vi "Config TDMS File for Asynchronous Write.vi"(8 "error in (no error)":errorcluster, 10 "rx channels":T1={"rx config"={"channel configuration"=[], "transfer mode"=enum."Finite", "sample rate"=10000000.0, "number of samples"=8192, "start trigger"=enum."Immediate"}, "reference frequency source"="Internal", "rx.data sink"=enum."Host", "rx.enabled channels"=[], "vertical range"=[], "rx.coerced configurations"={"coerced frequencies"=[], "coerced lo frequencies"=[], "coerced levels"=[], "coerced sample rates"=[]}} {"rx.coerced configurations"."coerced sample rates" format="%#.3pS/s"; "rx.coerced configurations"."coerced levels" format="%#.3gdBm"; "rx.coerced configurations"."coerced lo frequencies" format="%#.3pHz"; "rx.coerced configurations"."coerced frequencies" format="%#.3pHz"; "rx config"."channel configuration"."channel configuration"."frequency" format="%#.3pHz"; "rx config"."channel configuration"."channel configuration"."lo frequency" format="%#.3pHz"; "rx config"."channel configuration"."channel configuration"."level" format="%#_gdBm"; "rx config"."sample rate" format="%#.3pS/s"; "vertical range" format="%#.3pVpp"}, 11 "base path":path=path "D:/USRP Project TDMS Files") -> (0 "error out":errorcluster, 3 "Refnums out":refnum<k34>[](array[refnum]))   [LabVIEW 2016]
doc: "Configure TDMS Settings for asynchronous write"
uses:
  2954/SubVIs/Rx Channels.ctl
  2954/SubVIs/Start Trigger.ctl
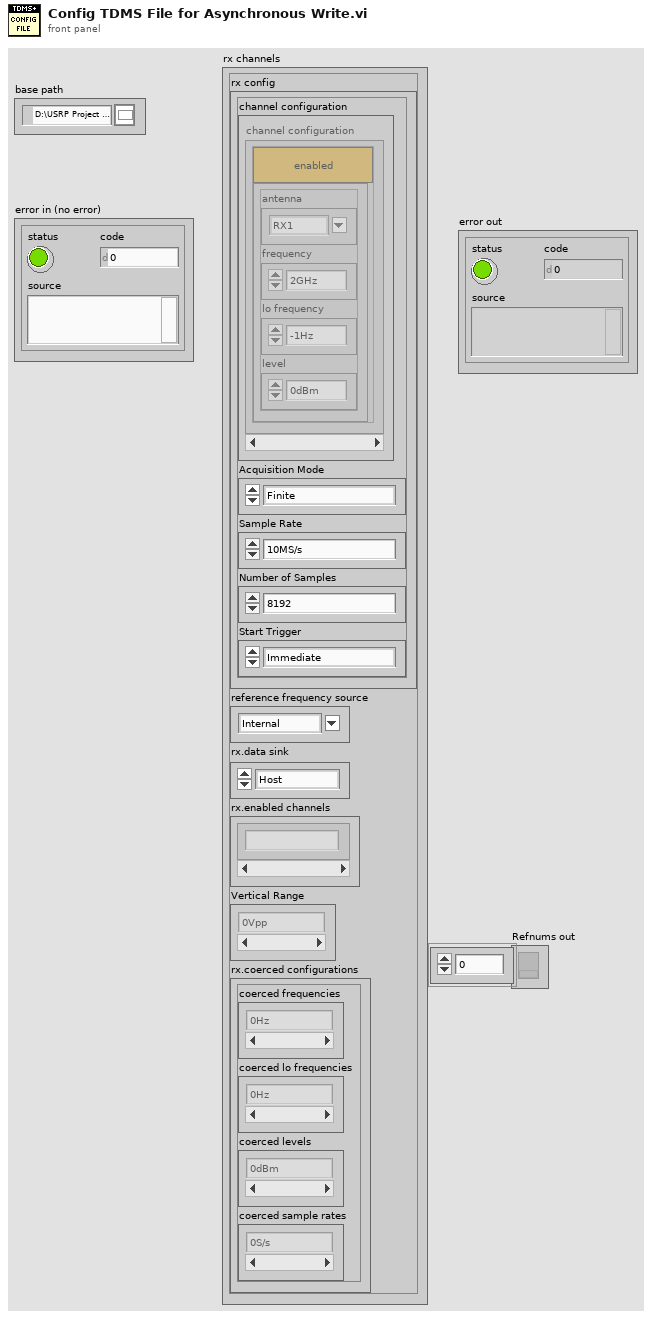
[diagram p1: front panel]
types:
  T1 = typedef "Rx Channels.ctl" = cluster{"rx config":cluster{"channel configuration":cluster{"channel enable":bool, "channel configuration":cluster{"antenna":string, "frequency":dbl, "lo frequency":dbl, "level":dbl}}[], "transfer mode":enum16{"Finite", "Continuous"}, "sample rate":dbl, "number of samples":u32, "start trigger":T2}, "reference frequency source":string, "rx.data sink":enum16{"SFP Port 0", "SFP Port 1", "Host"}, "rx.enabled channels":string[], "vertical range":dbl[], "rx.coerced configurations":cluster{"coerced frequencies":dbl[], "coerced lo frequencies":dbl[], "coerced levels":dbl[], "coerced sample rates":dbl[]}}
  T2 = typedef "Start Trigger.ctl" = enum8{"Software", "Digital Edge", "Rx Start Trigger", "Tx Start Trigger", "Immediate", "Future Time Event"}
  T3 = enum16{"open", "open or create", "create or replace", "create", "open (read-only)"}
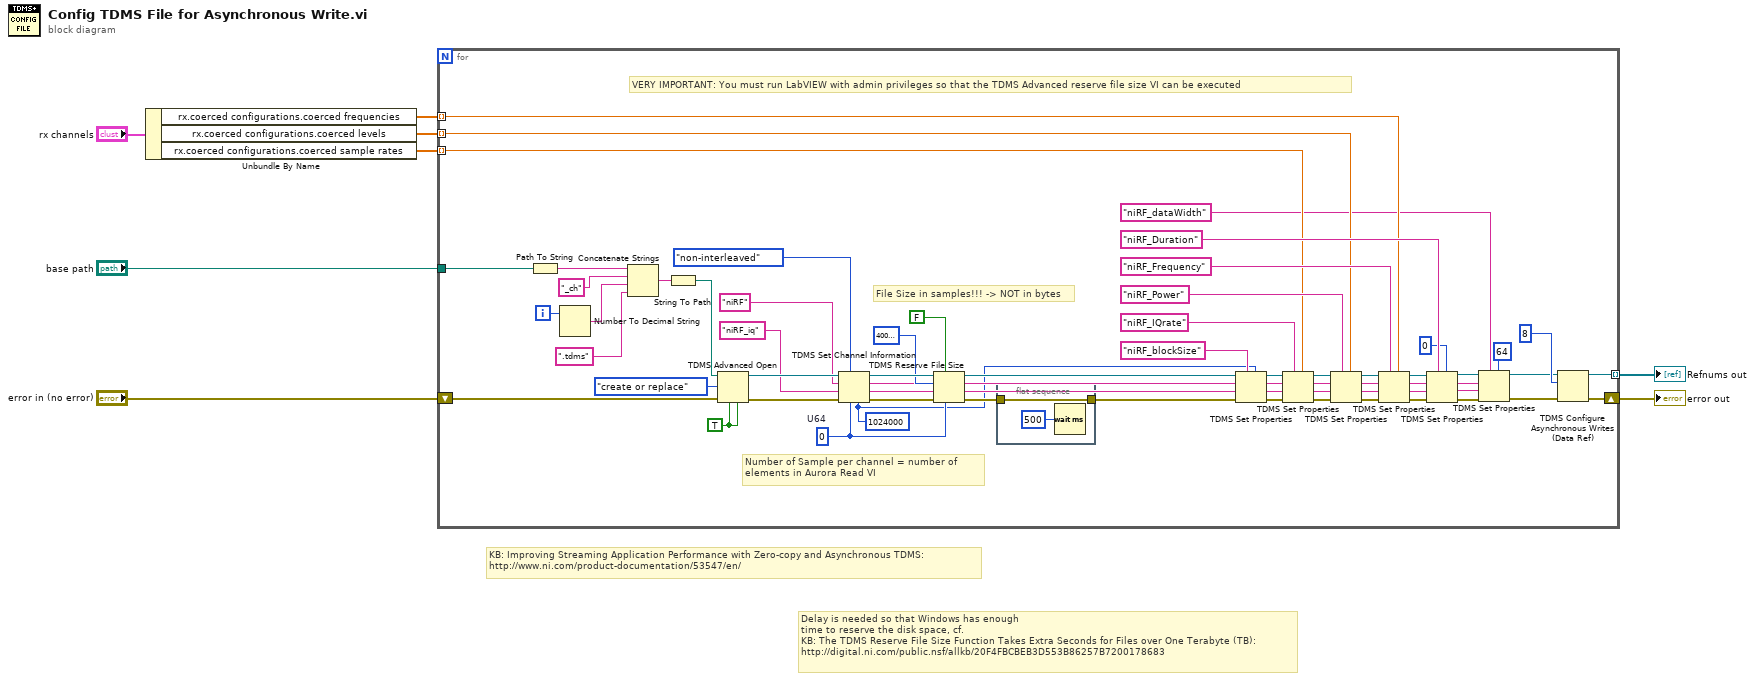
[diagram p0: block diagram]
diagram:
  # "KB: Improving Streaming Application Performance with Zero-copy and Asynchronous TDMS:\nhttp://www.ni.com/product-documentation/53547/en/"
  # "Delay is needed so that Windows has enough \ntime to reserve the disk space, cf.\nKB: The TDMS Reserve File Size Function Takes Extra Seconds for Files over One Terabyte (TB): \nhttp://digital.ni.com/public.nsf/allkb/20F4FBCBEB3D553B86257B7200178683"
  n1 = Unbundle By Name("rx channels") -> ("rx.coerced configurations.coerced frequencies"=w5:dbl[], "rx.coerced configurations.coerced levels"=w4:dbl[], "rx.coerced configurations.coerced sample rates"=w3:dbl[])
  n2 = for {
    shift-right: [w68] -> w8
    shift-left: "error in (no error)" -> [w60]
    tunnel: w5 -> [w32] mode=indexing
    tunnel: w4 -> [w31] mode=indexing
    tunnel: w3 -> [w30] mode=indexing
    tunnel: "base path" -> [w15]
    tunnel: [w11] -> w1 mode=indexing
    i -> [w13]
    w34 = "niRF_iq"
    w35 = "niRF"
    w20 = u32 1024000 ("samples per channel")
    w67 = u64 0  # U64
    w66 = TRUE ("enable asynchronous? (T)")
    # "File Size in samples!!! -> NOT in bytes"
    # "VERY IMPORTANT: You must run LabVIEW with admin privileges so that the TDMS Advanced reserve file size VI can be executed"
    # "Number of Sample per channel = number of \nelements in Aurora Read VI"
    n3 = Path To String(path=w15) -> (string=w16:string)
    n4 = Number To Decimal String(number=w13) -> (decimal integer string=w14:string)  [unwired: 1 in]
    n5 = Concatenate Strings(w16, "_ch" ("string"), w14, ".tdms" ("string")) -> (w18:string)
    n6 = String To Path(string=w18) -> (path=w12:path)
    n7 = TDMS Advanced Open(4:w66, 6:w66, 8:w60, 10:T3."create or replace" ("operation (0:open)"), 11:w12) -> (0:w61:errorcluster, 3:w62:refnum<k34>)  [unwired: 1 out]
    n8 = TDMS Set Channel Information(4:w20, 6:w67, 7:enum16{"non-interleaved", "interleaved"}."non-interleaved" ("data layout (0:non-interleaved)"), 8:w61, 9:w34, 10:w35, 11:w62) -> (0:w64:errorcluster, 3:w65:refnum<k34>)
    n9 = TDMS Reserve File Size(6:w67, 7:FALSE ("append? (T)"), 8:w64, 10:u64 40000000000 ("reserve size"), 11:w65) -> (0:w58:errorcluster, 3:w44:refnum<k34>)
    n10 = flat-sequence {
      tunnel: w58 -> [w71]
      tunnel: [w71] -> w33
      frame #0 {
        n11 = Wait (ms)(milliseconds to wait=u32 500) -> ()  [unwired: 1 out]
      }
    }
    n12 = TDMS Set Properties(5:w20, 7:"niRF_blockSize", 8:w33, 9:w34, 10:w35, 11:w44) -> (0:w42:errorcluster, 1:w40:string, 2:w41:string, 3:w43:refnum<k34>)
    n13 = TDMS Set Properties(5:w30, 7:"niRF_IQrate", 8:w42, 9:w40, 10:w41, 11:w43) -> (0:w56:errorcluster, 1:w55:string, 2:w54:string, 3:w53:refnum<k34>)
    n14 = TDMS Set Properties(5:w31, 7:"niRF_Power", 8:w56, 9:w55, 10:w54, 11:w53) -> (0:w52:errorcluster, 1:w51:string, 2:w50:string, 3:w49:refnum<k34>)
    n15 = TDMS Set Properties(5:w32, 7:"niRF_Frequency", 8:w52, 9:w51, 10:w50, 11:w49) -> (0:w48:errorcluster, 1:w47:string, 2:w46:string, 3:w45:refnum<k34>)
    n16 = TDMS Set Properties(5:u32 0 ("number of buffers (4)"), 7:"niRF_Duration", 8:w48, 9:w47, 10:w46, 11:w45) -> (0:w27:errorcluster, 1:w28:string, 2:w29:string, 3:w26:refnum<k34>)
    n17 = TDMS Set Properties(5:u32 64 ("number of buffers (4)"), 7:"niRF_dataWidth", 8:w27, 9:w28, 10:w29, 11:w26) -> (0:w24:errorcluster, 3:w25:refnum<k34>)  [unwired: 2 out]
    n18 = TDMS Configure Asynchronous Writes (Data Ref)(8:w24, 10:u32 8 ("number of buffers (4)"), 11:w25) -> (0:w68:errorcluster, 3:w11:refnum<k34>)  [unwired: 1 in]
  }
  "error out" <- w8
  "Refnums out" <- w1
